vi "Array 11.vi"() -> ()   [LabVIEW 2025]
panel:
  out "Array 3":dbl[](array[numeric])
  in  "Array 2":dbl[](array[numeric])
  in  "Array":dbl[](array[numeric])
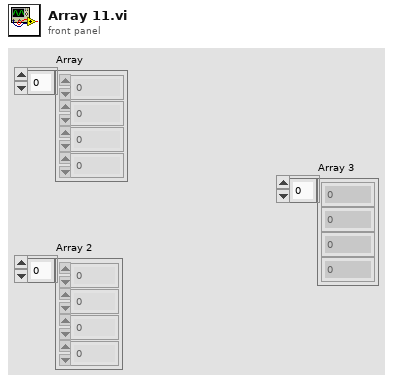
[diagram p1: front panel]
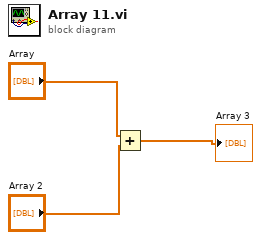
[diagram p0: block diagram]
diagram:
  n1 = Add(x="Array", y="Array 2") -> (x+y=→"Array 3":dbl[])
